vi "GA_Select.vi"(10 "fitness(500)_1":dbl[](array[numeric])) -> (0 "max index(es)":i32, 2 "pop[idx]_500":i32[](array[numeric]))   [LabVIEW 2018]
uses:
  GA_Global.vi
panel:
  out "32bit integer":i32[](array[numeric])
  out "x*y":dbl[](array[numeric])
  out "min index(es)":i32
  out "max index(es) 2":i32
  out "max value":dbl
  out "min value":dbl
  out "size(s)":i32
  out "Numeric":i32
  out "Array":i32[](array[numeric])
  out "x/y":dbl[](array[numeric])
  out "sum":dbl
  out "Array (Value)":i32[](array[numeric])
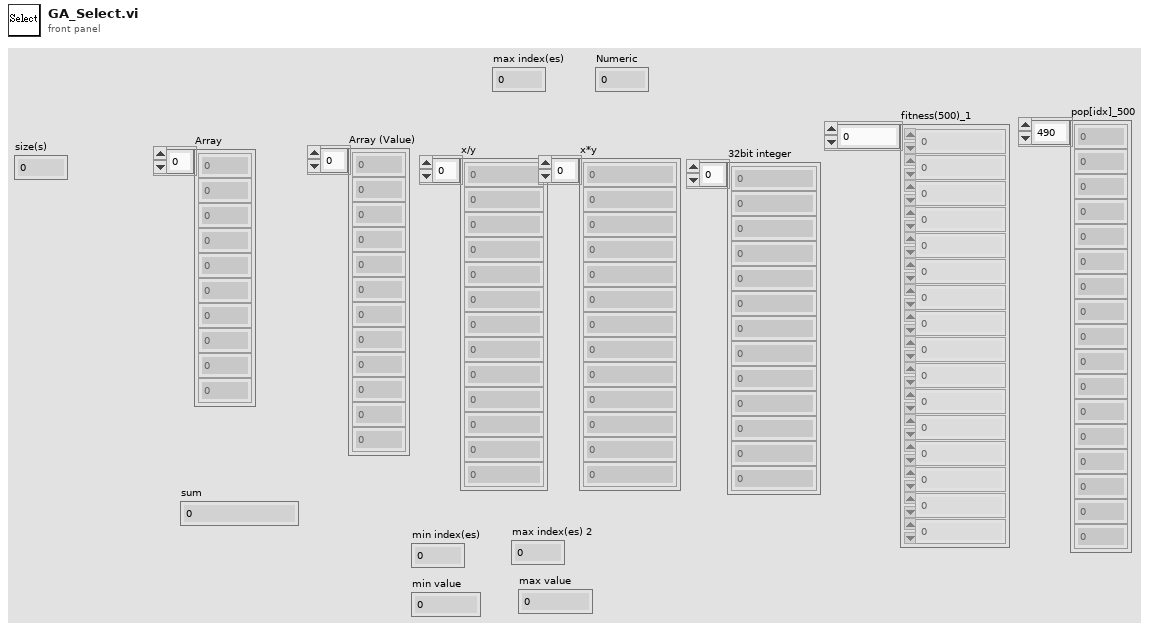
[diagram p1: front panel]
types:
  T1 = typedef "GA_parameter.ctl" = cluster{"N_CITIES":i32, "POP_SIZE":i32, "N_GENERATIONS":i32, "CROSS_RATE":dbl, "MUTATE_RATE":dbl}
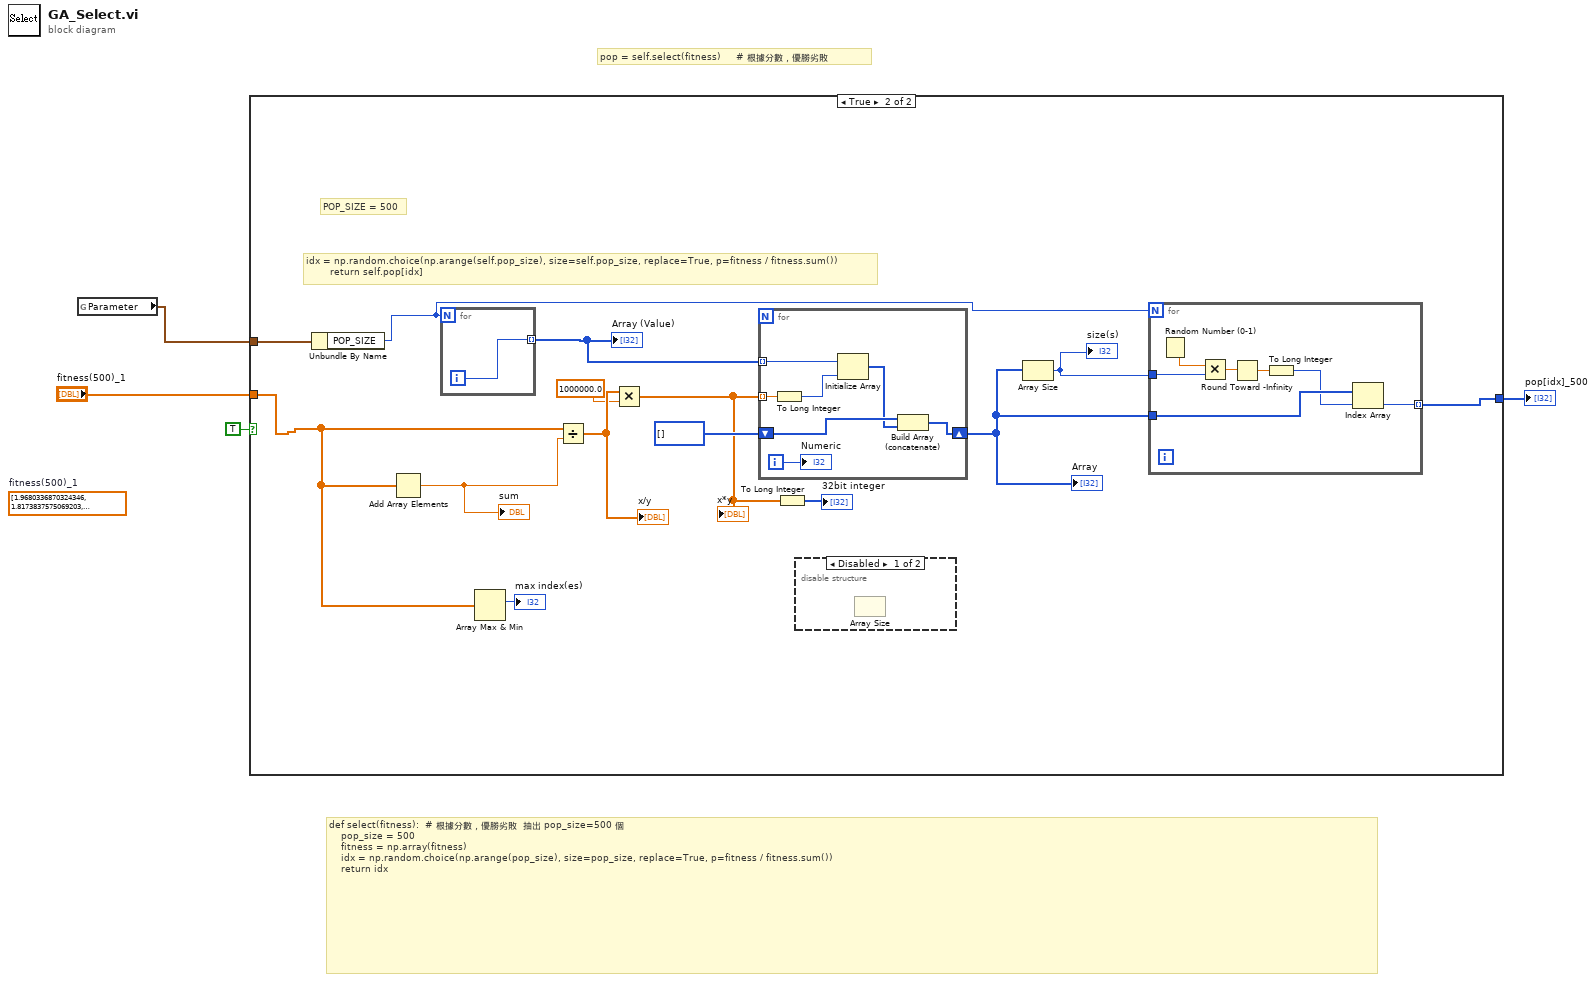
[diagram p0: block diagram]
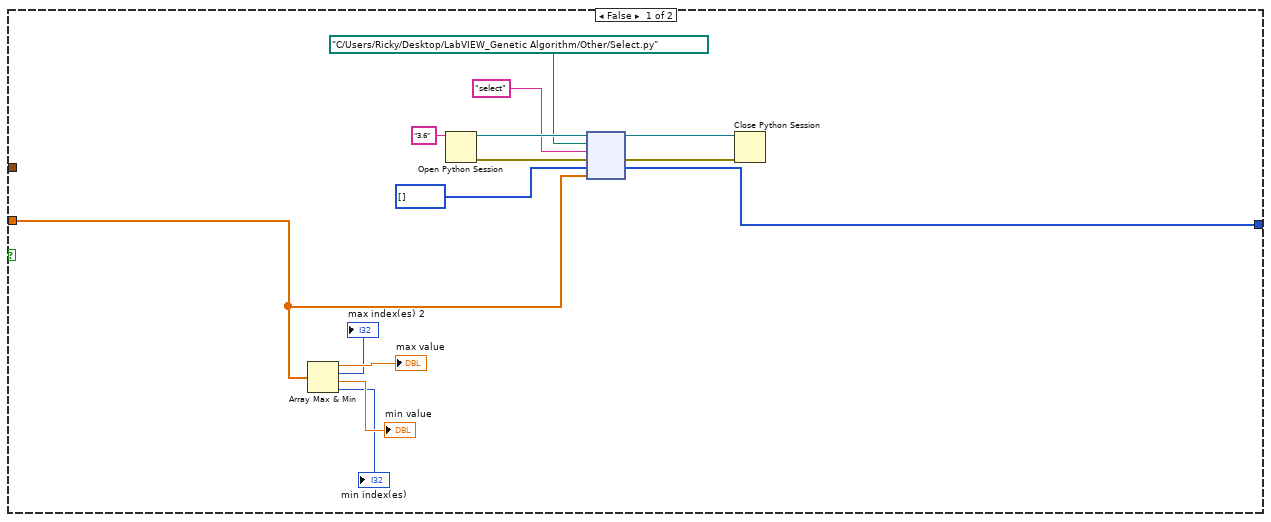
[diagram p2: hidden frame]
diagram:
  (unwired) dbl[] [1.9680336870324346, 1.8173837575069203, 1.9493133979419408, 2.0537900354011343, 1.700268821536934, 3.0576907557604422, 1.662032866371807, 1.8547110998509697, 1.7801736842997007, 2.112479528736684, 2.3429888654013933, 1.8267240522524604, 2.0197249104235473, 1.831609259193315, 2.076061899105873, 2.215358536883553, 1.8308933236484082, 1.6934540903231565, 1.8389888600734345, 1.8173004312816583, 2.215358536883553, 2.2966361880141855, 1.650268886854147, 1.8547110998509697, 2.2233878507438476, 2.001272097618607, 2.1019971784060134, 1.7424861857498235, 1.7636187635489549, 1.7921025686419403, 1.7707777231513857, 1.8162757804749603, 1.7424861857498235, 1.8222030326523686, 1.6145263612251612, 1.9583618237450346, 1.831609259193315, 1.7707777231513857, 1.8160628161248655, 2.0299305450786695, 1.88685020034852, 1.6869509039200798, 1.820693831823077, 2.1394013910465715, 2.001272097618607, 1.7707777231513857, 1.9811101814912984, 1.8527249208718117, 1.6627697280945015, 1.8267240522524604, 1.7472900775008566, 2.3775304593837956, 1.7801736842997007, 2.065175668379416, 2.854040248503228, 1.7795809195339325, 2.051399919924246, 2.001272097618607, 1.8162757804749603, 2.000283013580256, 1.8757641555873954, 2.032038613956254, 1.7631213538752502, 1.6392349058026978, 2.076061899105873, 1.8944220065094128, 1.8162757804749603, 1.625988585558044, 2.2233878507438476, 3.0576907557604422, 1.9665266158589438, 1.6711346033418881, 1.9583618237450346, 1.7346979717390076, 1.7953230116442438, 1.6575480868330916, 1.6042151400767846, 1.8137165656483145, 1.8019728240232373, 1.8173837575069203, 1.852812465650727, 2.0765962304743604, 1.63571139657188, 1.8272181976427322, 1.932444773338821, 1.8595118959751404, 1.8383264378907795, 1.960918053401361, 1.838759029187061, 2.1196418086014304, 1.7939339206254679, 1.7034137640238893, 1.959405406353109, 2.065175668379416, 1.7497718278564374, 2.1196418086014304, 2.0792004118325114, 1.8019728240232373, 1.5821961522354677, 2.075797635268095, 2.1196418086014304, 2.5268544053564312, 1.6704751932581607, 1.8595118959751404, 1.820693831823077, 1.9057099217555618, 1.7631213538752502, 1.6042151400767846, 2.0946090857291977, 1.7606311241427308, 1.982530666964055, 1.7801736842997007, 1.959405406353109, 2.5268544053564312, 1.7707777231513857, 2.5268544053564312, 2.141777687060943, 1.7077032707818387, 1.743553249236235, 1.7034137640238893, 1.6042151400767846, 2.1035527553823603, 2.2597560045257947, 2.253830132283526, 1.9853863782257248, 1.6531956923304338, 1.650268886854147, 2.276888358467702, 2.0397086322227485, 1.7636187635489549, 1.75911808290768, 1.752573073977762, 1.7034137640238893, 1.8222030326523686, 1.7482152296809124, 1.7875390572469547, 1.6042151400767846, 1.782422203020611, 2.0130586901436707, 2.074016751296446, 2.0130586901436707, 1.7616371975964964, 1.8086750791964246, 1.8086750791964246, 1.8647208011765675, 2.057116074950381, 1.8383264378907795, 3.0066856640185606, 2.000283013580256, 1.75911808290768, 1.71252760968179, 1.7346979717390076, 1.835682615469146, 1.832066608352659, 1.7631213538752502, 2.0765962304743604, 1.6869509039200798, 2.1337962866602593, 1.752573073977762, 1.7324133732211726, 1.9665266158589438, 1.7790203508914337, 1.7472900775008566, 2.075797635268095, 2.2233878507438476, 1.9487057837079176, 1.7647982169216172, 2.402919817573543, 1.732472540138863, 1.9102050595102424, 1.6805847359588155, 1.8547110998509697, 1.7346979717390076, 1.7572909427511008, 2.4079605392159316, 2.000283013580256, 1.6627697280945015, 1.7864340892312158, 1.7636187635489549, 2.2966361880141855, 1.5821961522354677, 1.6627697280945015, 1.7953230116442438, 1.9493133979419408, 1.6576342901814063, 1.7864340892312158, 1.852812465650727, 1.7875390572469547, 1.8464250641201694, 2.0397086322227485, 1.8944220065094128, 1.7498078974716125, 2.0334999056282723, 2.1035527553823603, 1.6686861194523117, 1.637951717773023, 3.0066856640185606, 1.6575480868330916, 2.3429888654013933, 2.0299305450786695, 1.6934540903231565, 2.033696583362432, 2.0537900354011343, 1.743553249236235, 2.001272097618607, 2.854040248503228, 1.7346979717390076, 1.9493133979419408, 1.6686861194523117, 2.074016751296446, 1.7409236583609196, 2.371710328263902, 1.700268821536934, 1.832066608352659, 2.001272097618607, 1.8944220065094128, 1.9680336870324346, 1.7424861857498235, 2.0792004118325114, 1.7497718278564374, 2.065175668379416, 1.71252760968179, 1.8086750791964246, 2.2966361880141855, 1.9487057837079176, 2.0334999056282723, 1.9886631568587703, 1.838759029187061, 1.9853863782257248, 2.335312985422951, 2.253830132283526, 1.7616371975964964, 1.7077032707818387, 2.4699944997884815, 1.8647208011765675, 1.7497718278564374, 2.2966361880141855, 1.6531956923304338, 1.959405406353109, 2.3603481658316516, 1.732472540138863, 2.032038613956254, 2.000283013580256, 1.6934540903231565, 1.7616371975964964, 1.7409236583609196, 1.6392349058026978, 1.6576342901814063, 1.9057099217555618, 1.7953230116442438, 2.72310081816729, 2.854040248503228, 1.835682615469146, 1.8162757804749603, 1.8652889295708255, 2.0946090857291977, 2.0397086322227485, 1.9886631568587703, 1.8160628161248655, 2.0130586901436707, 1.732472540138863, 3.0576907557604422, 1.9232054704137607, 1.9583618237450346, 1.7939339206254679, 2.0537900354011343, 1.7707777231513857, 1.75911808290768, 2.076061899105873, 1.7707777231513857, 2.402919817573543, 1.7953230116442438, 2.112479528736684, 1.8173837575069203, 1.8222030326523686, 2.473235129066634, 2.141777687060943, 1.743553249236235, 3.0066856640185606, 2.1337962866602593, 1.6934540903231565, 1.743553249236235, 1.7910684155204737, 1.7941744613386243, 1.6575480868330916, 1.9886631568587703, 2.001272097618607, 1.8207754138106846, 2.065175668379416, 1.7636187635489549, 1.6934540903231565, 1.9853863782257248, 1.8308933236484082, 2.2142460338614645, 2.0580844653901904, 2.051399919924246, 1.832066608352659, 2.72310081816729, 1.9665266158589438, 1.8134067862938457, 1.8006434420783253, 2.0765962304743604, 1.6042151400767846, 2.3603481658316516, 1.838759029187061, 2.266234157894476, 2.2142460338614645, 1.8389888600734345, 1.6805847359588155, 2.0792004118325114, 2.032038613956254, 1.7939339206254679, 1.8272181976427322, 1.6809301319467576, 2.569360347252037, 2.371710328263902, 2.076061899105873, 1.7939339206254679, 1.7549819399663544, 1.7482152296809124, 2.253830132283526, 2.266234157894476, 1.8464250641201694, 2.402919817573543, 1.932444773338821, 2.0237918367975487, 1.8137165656483145, 2.0580844653901904, 1.7713193940490215, 1.6481881201770856, 2.0299305450786695, 1.800304981805827, 1.9232054704137607, 1.730392720703012, 2.215358536883553, 2.0792004118325114, 1.8267240522524604, 1.6869509039200798, 2.0299305450786695, 1.7795809195339325, 1.832066608352659, 1.8308933236484082, 2.000283013580256, 1.776536538871944, 2.3775304593837956, 1.6042151400767846, 2.8203806297906215, 2.0792004118325114, 2.0792004118325114, 1.8584326782849256, 2.371710328263902, 1.7572909427511008, 3.0066856640185606, 1.982530666964055, 1.9886631568587703, 1.6734050039184483, 2.0197249104235473, 1.7801736842997007, 2.065175668379416, 1.838759029187061, 2.2597560045257947, 2.854040248503228, 1.7790203508914337, 1.8006434420783253, 2.0197249104235473, 1.718888405605394, 1.7953230116442438, 1.7175594313635847, 1.7713193940490215, 2.854040248503228, 2.032038613956254, 1.730392720703012, 1.8173004312816583, 2.0197249104235473, 1.9886631568587703, 2.253830132283526, 1.7939339206254679, 1.6392349058026978, 1.8173837575069203, 1.732472540138863, 2.0130586901436707, 1.6805847359588155, 2.1394013910465715, 2.335312985422951, 2.001272097618607, 1.6663875633087344, 2.1196418086014304, 1.8173837575069203, 2.327058773512028, 1.7520608415347785, 1.8019728240232373, 1.8019728240232373, 2.8203806297906215, 1.700268821536934, 1.8724693622544977, 2.000283013580256, 2.8801881481069778, 1.8389888600734345, 1.9493133979419408, 1.9665266158589438, 1.838759029187061, 2.3603481658316516, 2.3429888654013933, 2.4699944997884815, 1.7616371975964964, 2.001272097618607, 2.854040248503228, 1.6734050039184483, 1.9853863782257248, 1.8724693622544977, 2.0884501431691582, 1.9997142546653246, 2.3603481658316516, 1.8595118959751404, 1.9487057837079176, 2.5268544053564312, 2.276888358467702, 1.7631213538752502, 1.6481881201770856, 1.7795809195339325, 2.0130586901436707, 1.7921025686419403, 1.752573073977762, 2.72310081816729, 1.831609259193315, 1.662032866371807, 1.820693831823077, 1.7606311241427308, 2.3775304593837956, 2.0765962304743604, 2.276888358467702, 1.8160628161248655, 1.8162757804749603, 1.9886631568587703, 1.9997142546653246, 1.7175594313635847, 2.3603481658316516, 1.7921025686419403, 1.7549819399663544, 2.335312985422951, 3.0576907557604422, 1.7864340892312158, 1.7034137640238893, 1.8272181976427322, 2.335312985422951, 1.8267240522524604, 1.6934540903231565, 1.732472540138863, 1.8267240522524604, 2.0299305450786695, 1.7472900775008566, 2.2597560045257947, 3.0066856640185606, 2.1337962866602593, 1.6809301319467576, 1.9886631568587703, 1.7875390572469547, 2.2142460338614645, 2.0197249104235473, 1.63571139657188, 1.8207754138106846, 1.7864340892312158, 1.8780096709798677, 1.7346979717390076, 1.7472900775008566, 1.650268886854147, 1.6392349058026978, 2.215358536883553, 2.0765962304743604, 2.277729558447695, 1.6392349058026978, 1.8222030326523686, 1.9997142546653246, 1.718888405605394, 1.835682615469146, 1.6576342901814063, 2.3603481658316516, 1.6392349058026978, 1.7324133732211726, 1.6936242653085736, 1.7498894134809837, 1.8267240522524604, 1.7975257179552837, 1.6869509039200798, 1.634576875540678, 2.276888358467702, 2.253830132283526, 2.289285777756575, 1.8173837575069203, 1.7346979717390076, 1.7034137640238893, 1.7497718278564374, 1.6704751932581607, 1.7795809195339325, 2.266234157894476, 2.1035527553823603, 1.7498894134809837, 1.959405406353109, 2.3429888654013933, 1.732472540138863]  # fitness(500)_1
  # "def select(fitness):  # 根據分數，優勝劣敗  抽出 pop_size=500 個\n    pop_size = 500\n    fitness = np.array(fitness)\n    idx = np.random.choice(np.arange(pop_size), size=pop_size, replace=True, p=fitness / fitness.sum())\n    return idx"
  # "pop = self.select(fitness)     # 根據分數，優勝劣敗"
  n1 = global read "GA_Global.vi" "Parameter"() -> (w4:T1)
  n2 = case shown="True" TRUE {
    tunnel: w4 -> [_ w32]
    tunnel: [w10 w23] -> w3
    tunnel: "fitness(500)_1" -> [w9 w22]
    frame False {
      n3 = Array Max & Min(array=w9) -> (max value=→"max value":dbl, max index (indices)=→"max index(es) 2":i32, min value=→"min value":dbl, min index (indices)=→"min index(es)":i32)
      n4 = Open Python Session(python version="3.6" ("Python version")) -> (session out=w18:refnum<k35>, error out=w15:errorcluster)  [unwired: 2 in]
      n5 = node(w18, path "C:/Users/Ricky/Desktop/LabVIEW_Genetic Algorithm/Other/Select.py" ("module path"), "select" ("function name"), w15, i32[] [], w9) -> (w17:refnum<k35>, w14:errorcluster, w10:i32[])  [unwired: 1 in, 2 out]
      n6 = Close Python Session(session in=w17, error in=w14) -> ()  [unwired: 1 out]
    }
    frame True {
      # "POP_SIZE = 500"
      # "idx = np.random.choice(np.arange(self.pop_size), size=self.pop_size, replace=True, p=fitness / fitness.sum())\n        return self.pop[idx]"
      n7 = Unbundle By Name(w32) -> ("POP_SIZE"=w26:i32)
      n8 = Add Array Elements(numeric array=w22) -> (sum=w31:dbl)
      "sum" <- w31
      n9 = for {
        N: w26 -> [_]
        tunnel: [w47] -> w28 mode=indexing
        i -> [w47]
      }
      "Array (Value)" <- w28
      n10 = Array Max & Min(array=w22) -> (max index (indices)=→"max index(es)":i32)  [unwired: 3 out]
      n11 = Divide(x=w22, y=w31) -> (x/y=w30:dbl[])
      "x/y" <- w30
      n12 = Multiply(x=w30, y=1000000.0) -> (x*y=w20:dbl[])
      "x*y" <- w20
      n13 = for {
        tunnel: w28 -> [w42] mode=indexing
        tunnel: w20 -> [w44] mode=indexing
        shift-right: [w45] -> w25
        shift-left: i32[] [] -> [w46]
        i -> [w40]
        n14 = To Long Integer(number=w44) -> (32bit integer=w43:i32)
        n15 = Initialize Array(w42, w43) -> (w41:i32[])
        n16 = Build Array (concatenate)(w46, w41) -> (w45:i32[])
        "Numeric" <- w40
      }
      "Array" <- w25
      n17 = To Long Integer(number=w20) -> (32bit integer=→"32bit integer":i32[])
      n18 = disable-structure shown="Disabled" {
        frame Disabled {
          n19 = Array Size() -> ()  [unwired: 1 in, 1 out]
        }
        frame Enabled {
        }
      }
      n20 = Array Size(array=w25) -> (size(s)=w24:i32)
      "size(s)" <- w24
      n21 = for {
        N: w26 -> [_]
        tunnel: w25 -> [w37]
        tunnel: w24 -> [w38]
        tunnel: [w36] -> w23 mode=indexing
        n22 = Random Number (0-1)() -> (number: 0 to 1=w35:dbl)
        n23 = Multiply(x=w35, y=w38) -> (x*y=w39:dbl)
        n24 = Round Toward -Infinity(1:w39) -> (0:w34:dbl)
        n25 = To Long Integer(number=w34) -> (32bit integer=w33:i32)
        n26 = Index Array(array=w37, index=w33) -> (element=w36:i32)
      }
    }
  }
  "pop[idx]_500" <- w3
